vi "VI_CheckIfChExists.vi"(8 "error in (no error)":errorcluster, 10 "Channel Name To Check":string, 11 "ChList_Ref In":refnum<vi>) -> (0 "error out":errorcluster, 2 "Channel Exists":bool, 3 "ChList_Ref Out":refnum<vi>)   [LabVIEW 2018]
panel:
  in  "LBox_ChList":i32(listbox)
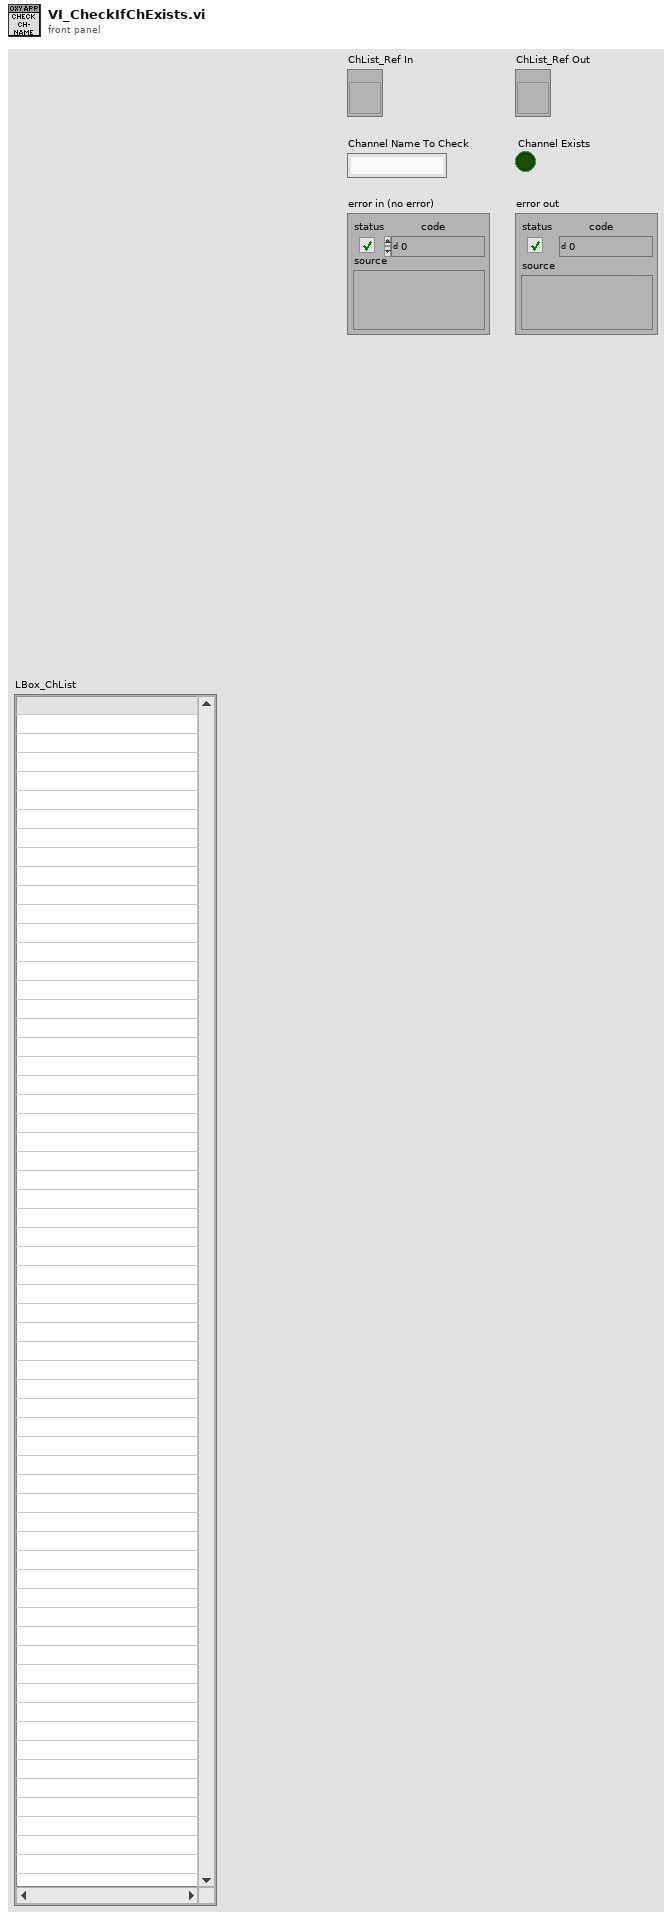
[diagram p1: front panel]
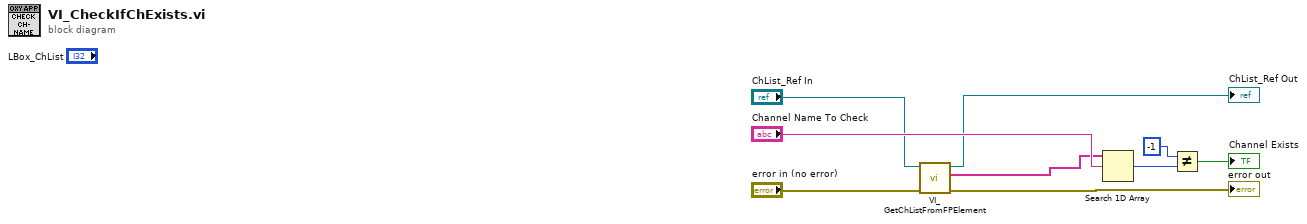
[diagram p0: block diagram]
diagram:
  n1 = call "VI_GetChListFromFPElement.vi"("error in (no error)"="error in (no error)", "ChList_Ref In"="ChList_Ref In") -> ("error out"=→"error out":errorcluster, "Channel Names"=w4:string[], "ChList_Ref Out"=→"ChList_Ref Out":refnum<vi>)  [unwired: 6 in, 1 out]
  n2 = Search 1D Array(1D array=w4, element="Channel Name To Check") -> (index of element=w3:i32)  [unwired: 1 in]
  n3 = Not Equal?(x=-1, y=w3) -> (x != y?=→"Channel Exists":bool)
